vi "Disconnect SMU Resources from site - Site SMUs only.vi"(0 "TSM context":T1, 11 "error in":errorcluster) -> (4 "TSM context out":T1, 15 "error out":errorcluster)   [LabVIEW 2019]
doc: "This VI is used to disconnect SMU resources safely by preventing potetial OCP errors."
uses:
  <vilib>/NI_TestStand_SemiconductorModule/NI_TestStand_Semiconductor_Module.lvlibp/PinMap/General/SemiconductorModuleContext.ctl
  <instrlib>/niDCPower/nidcpower.llb/niDCPower Output Function.ctl
  <instrlib>/niDCPower/nidcpower.llb/niDCPower Sense.ctl
  <instrlib>/niDCPower/nidcpower.llb/niDCPower Source Mode.ctl
  TSM Context Data Access/Public/Properties/TestFlowID - Read.vi
  <vilib>/NI_TestStand_SemiconductorModule/NI_TestStand_Semiconductor_Module.lvlibp
  TSM Context Data Access/TSM Context Data Access.lvclass
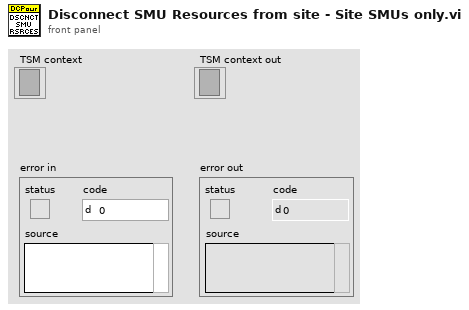
[diagram p1: front panel]
types:
  T1 = typedef "NI_TestStand_Semiconductor_Module.lvlibp/SemiconductorModuleContext.ctl" = refnum<k7>
  T2 = typedef "niDCPower Source Mode.ctl" = i32
  T3 = typedef "niDCPower Sense.ctl" = i32
  T4 = typedef "niDCPower Output Function.ctl" = i32
  T5 = typedef "TSM SSC DCPower.ctl" = cluster{"Pin Query Context":refnum<class "MultiplePinMultipleSessionQueryContext.lvclass">, "SSC":T6[], "Site Numbers":i32[], "Pins":T7[], "Pins Expanded":T9[]}
  T6 = typedef "SSC DCPower.ctl" = cluster{"Session":refnum<k15>, "Chan":string, "Channel List":string}
  T7 = typedef "TSM Pin Information.ctl" = cluster{"Pin":tag, "Type":T8, "Count":i32}
  T8 = typedef "TSM Pin Type Identifier.ctl" = enum8{"DUT Pin", "System Pin", "Pin Group", "Not Determined"}
  T9 = typedef "TSM Expanded Pin Information.ctl" = cluster{"Pin":tag, "Type":T8, "Index":i32}
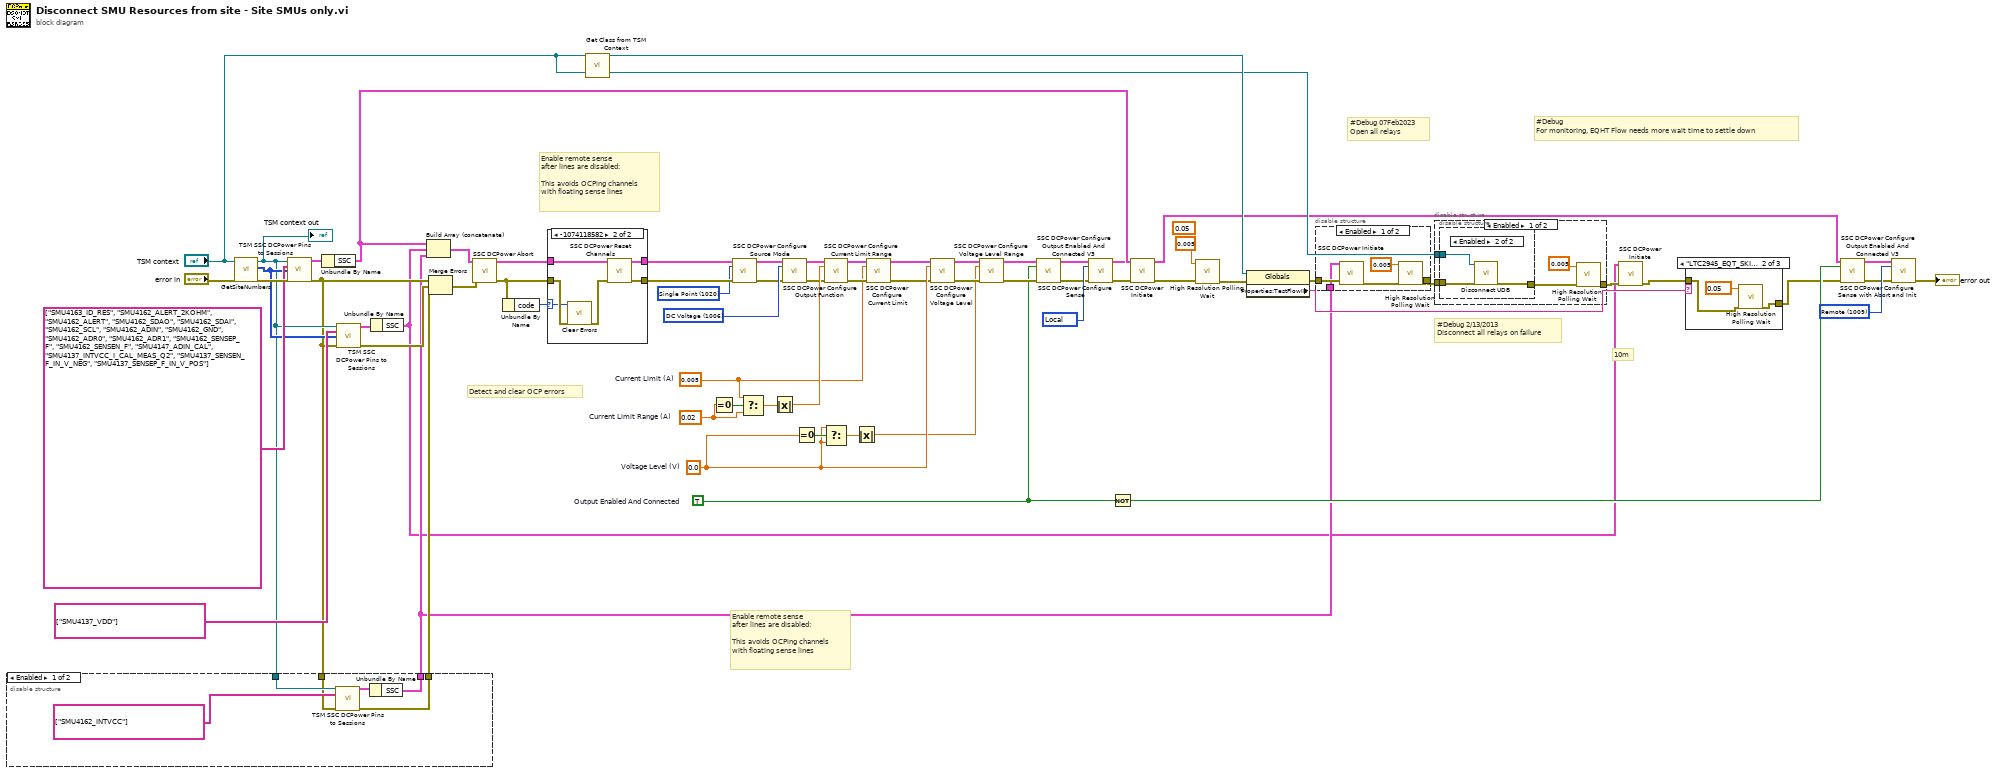
[diagram p0: block diagram]
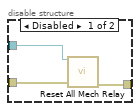
[diagram p2: hidden frame]
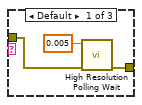
[diagram p6: hidden frame]
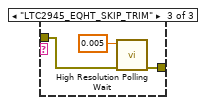
[diagram p7: hidden frame]
diagram:
  (unwired) 0.05 ("seconds to wait")
  w36 = T2 1020 items=["Single Point"=1020, "Sequence"=1021] ("Source Mode")
  w41 = T3 1009 items=["Local"=1008, "Remote"=1009] ("Sense")
  w43 = T3 1008 items=["Local"=1008, "Remote"=1009] ("Sense")
  w52 = T4 1006 items=["DC Voltage"=1006, "DC Current"=1007, "Pulse Voltage"=1049, "Pulse Current"=1050] ("Output Function")
  w51 = 0.005  # Current Limit (A)
  w49 = 0.0  # Voltage Level (V)
  w50 = 0.02  # Current Limit Range (A)
  w31 = TRUE  # Output Enabled And Connected
  # "10m"
  # "#Debug 2/13/2013\nDisconnect all relays on failure"
  # "#Debug 07Feb2023\nOpen all relays"
  # "#Debug\nFor monitoring, EQHT Flow needs more wait time to settle down"
  # "Enable remote sense\nafter lines are disabled:\n\nThis avoids OCPing channels\nwith floating sense lines"
  # "Enable remote sense\nafter lines are disabled:\n\nThis avoids OCPing channels\nwith floating sense lines"
  # "Detect and clear OCP errors"
  n1 = call <vilib>:"GetSiteNumbers.vi"("error in (no error)"="error in", "Semiconductor Module Context"="TSM context") -> ("error out"=w62:errorcluster, "Site Numbers"=w14:i32[], "Semiconductor Module Context Out"=w13:T1)  [unwired: 6 in, 1 out]
  "TSM context out" <- w13
  n2 = call "TSM SSC DCPower Pins to Sessions.vi"("TSM context"=w13, "Pins"=tag[] ["SMU4163_ID_RES", "SMU4162_ALERT_2KOHM", "SMU4162_ALERT", "SMU4162_SDAO", "SMU4162_SDAI", "SMU4162_SCL", "SMU4162_ADIN", "SMU4162_GND", "SMU4162_ADR0", "SMU4162_ADR1", "SMU4162_SENSEP_F", "SMU4162_SENSEN_F", "SMU4147_ADIN_CAL", "SMU4137_INTVCC_I_CAL_MEAS_Q2", "SMU4137_SENSEN_F_IN_V_NEG", "SMU4137_SENSEP_F_IN_V_POS"], "Site Numbers"=w14, "error in"=w62) -> ("DCPower TSM Out"=w64:T5, "error out"=w12:errorcluster)  [unwired: 10 in]
  n3 = disable-structure shown="Enabled" {
    disable-tunnel: w13 -> [w71 _]
    disable-tunnel: w12 -> [w69 _]
    disable-tunnel: [w68 _] -> w11
    disable-tunnel: [w67 _] -> w10
    frame Enabled {
      n4 = call "TSM SSC DCPower Pins to Sessions.vi"("TSM context"=w71, "Pins"=tag[] ["SMU4162_INTVCC"] ("Pin"), "error in"=w69) -> ("DCPower TSM Out"=w70:T5, "error out"=w68:errorcluster)  [unwired: 11 in]
      n5 = Unbundle By Name(w70) -> ("SSC"=w67:T6[])
    }
    frame Disabled {
    }
  }
  n6 = Unbundle By Name(w64) -> ("SSC"=w21:T6[])
  n7 = call "TSM SSC DCPower Pins to Sessions.vi"("TSM context"=w13, "Pins"=tag[] ["SMU4137_VDD"] ("Pin"), "Site Numbers"=w14, "error in"=w12) -> ("DCPower TSM Out"=w23:T5, "error out"=w25:errorcluster)  [unwired: 10 in]
  n8 = Unbundle By Name(w23) -> ("SSC"=w2:T6[])
  n9 = Build Array (concatenate)(w21, w2, w10) -> (w22:T6[])
  n10 = Merge Errors(w12, w25, w11) -> (w24:errorcluster)
  n11 = call "SSC DCPower Abort.vi"("DCPower SSC in"=w22, "error in"=w24) -> ("DCPower SSC out"=w63:T6[], "error out"=w65:errorcluster)  [unwired: 12 in]
  n12 = Unbundle By Name(w65) -> ("code"=w66:i32)
  n13 = case shown="-1074118582" w66 {
    selector: w66 -> [_ w77]
    tunnel: [w74 w79] -> w40
    tunnel: w65 -> [w74 w80]
    tunnel: w63 -> [w73 w76]
    tunnel: [w73 w75] -> w39
    frame Default {
    }
    frame -1074118582 {
      n14 = call <vilib>:"Clear Errors.vi"("error in (no error)"=w80, "specific error code to clear (0: all)"=w77) -> ("error out"=w78:errorcluster)  [unwired: 4 in, 1 out]
      n15 = call "SSC DCPower Reset Channels.vi"("DCPower SSC in"=w76, "error in"=w78) -> ("DCPower SSC out"=w75:T6[], "error out"=w79:errorcluster)  [unwired: 12 in]
    }
  }
  n16 = call "Get Class from TSM Context.vi"("TSM Context"="TSM context") -> ("Global Memory Class"=w18:refnum<class "TSM Context Data Access.lvclass">)  [unwired: 14 in]
  n17 = Equal To 0?(x=w50) -> (x = 0?=w60:bool)
  n18 = call "SSC DCPower Configure Source Mode.vi"("DCPower SSC in"=w39, "Source Mode"=w36, "error in"=w40) -> ("DCPower SSC out"=w37:T6[], "error out"=w38:errorcluster)  [unwired: 11 in]
  n19 = Select(t=w51, s=w60, f=w50) -> (s? t:f=w59:dbl)
  n20 = Absolute Value(x=w59) -> (abs(x)=w61:dbl)
  n21 = call "SSC DCPower Configure Output Function.vi"("DCPower SSC in"=w37, "Output Function"=w52, "error in"=w38) -> ("DCPower SSC out"=w53:T6[], "error out"=w54:errorcluster)  [unwired: 11 in]
  n22 = Equal To 0?(x=w49) -> (x = 0?=w57:bool)
  n23 = call "SSC DCPower Configure Current Limit Range.vi"("DCPower SSC in"=w53, "Current Limit Range (A)"=w61, "error in"=w54) -> ("DCPower SSC out"=w55:T6[], "error out"=w56:errorcluster)  [unwired: 11 in]
  n24 = Select(t=w49, s=w57, f=w49) -> (s? t:f=w58:dbl)
  n25 = Absolute Value(x=w58) -> (abs(x)=w44:dbl)
  n26 = call "SSC DCPower Configure Current Limit.vi"("DCPower SSC in"=w55, "Current Limit (A)"=w51, "error in"=w56) -> ("DCPower SSC out"=w47:T6[], "error out"=w48:errorcluster)  [unwired: 11 in]
  n27 = call "SSC DCPower Configure Voltage Level.vi"("DCPower SSC in"=w47, "Voltage Level (V)"=w49, "error in"=w48) -> ("DCPower SSC out"=w45:T6[], "error out"=w46:errorcluster)  [unwired: 11 in]
  n28 = call "SSC DCPower Configure Voltage Level Range.vi"("DCPower SSC in"=w45, "Voltage Level Range (V)"=w44, "error in"=w46) -> ("DCPower SSC out"=w32:T6[], "error out"=w33:errorcluster)  [unwired: 11 in]
  n29 = call "SSC DCPower Configure Output Enabled And Connected V3.vi"("DCPower SSC in"=w32, "Output Enabled And Connected"=w31, "error in"=w33) -> ("DCPower SSC out"=w29:T6[], "error out"=w30:errorcluster)  [unwired: 11 in]
  n30 = call "SSC DCPower Configure Sense.vi"("DCPower SSC in"=w29, "Sense"=w43, "error in"=w30) -> ("DCPower SSC out"=w8:T6[], "error out"=w42:errorcluster)  [unwired: 11 in]
  n31 = Not(x=w31) -> (.not. x?=w16:bool)
  n32 = call "SSC DCPower Initiate.vi"("DCPower SSC in"=w21, "error in"=w42) -> ("error out"=w7:errorcluster)  [unwired: 12 in, 1 out]
  n33 = call <vilib>:"High Resolution Polling Wait.vi"("error in (no error)"=w7, "seconds to wait"=0.005) -> ("error out"=w6:errorcluster)  [unwired: 9 in]
  n34 = property class="Globals"(reference=w18, error in=w6) -> (error out=w19:errorcluster, "Properties:TestFlowID"=w20:string)  [unwired: 1 out]
  n35 = disable-structure shown="Enabled" {
    disable-tunnel: w19 -> [w85 w86]
    disable-tunnel: w10 -> [w84 _]
    disable-tunnel: [w82 w86] -> w9
    frame Enabled {
      n36 = call "SSC DCPower Initiate.vi"("DCPower SSC in"=w84, "error in"=w85) -> ("error out"=w83:errorcluster)  [unwired: 12 in, 1 out]
      n37 = call <vilib>:"High Resolution Polling Wait.vi"("error in (no error)"=w83, "seconds to wait"=0.005) -> ("error out"=w82:errorcluster)  [unwired: 9 in]
    }
    frame Disabled {
    }
  }
  n38 = disable-structure shown="Enabled" {
    disable-tunnel: "TSM context" -> [w91 _]
    disable-tunnel: w9 -> [w90 w98]
    disable-tunnel: [w88 w98] -> w3
    frame Enabled {
      n39 = disable-structure shown="Enabled" {
        disable-tunnel: w90 -> [w94 w97]
        disable-tunnel: [w93 w96] -> w89
        disable-tunnel: w91 -> [w92 w95]
        frame Disabled {
          n40 = call "Reset All Mech Relay.vi"("TSM Context"=w92, "error in (no error)"=w94) -> ("error out"=w93:errorcluster)  [unwired: 13 in]
        }
        frame Enabled {
          n41 = call "Disconnect UDB.vi"("error in (no error)"=w97, "Semiconductor Module Context"=w95) -> ("error out"=w96:errorcluster)  [unwired: 9 in]
        }
      }
      n42 = call <vilib>:"High Resolution Polling Wait.vi"("error in (no error)"=w89, "seconds to wait"=0.005) -> ("error out"=w88:errorcluster)  [unwired: 9 in]
    }
    frame Disabled {
    }
  }
  n43 = call "SSC DCPower Initiate.vi"("DCPower SSC in"=w2, "error in"=w3) -> ("error out"=w1:errorcluster)  [unwired: 12 in, 1 out]
  n44 = case shown="\"LTC2945_EQT_SKIP_TRIM\"" w20 {
    tunnel: [w100 w102 w106] -> w4
    tunnel: w1 -> [w99 w103 w105]
    frame Default {
      n45 = call <vilib>:"High Resolution Polling Wait.vi"("error in (no error)"=w99, "seconds to wait"=0.005) -> ("error out"=w100:errorcluster)  [unwired: 9 in]
    }
    frame "LTC2945_EQT_SKIP_TRIM" {
      n46 = call <vilib>:"High Resolution Polling Wait.vi"("error in (no error)"=w103, "seconds to wait"=0.05) -> ("error out"=w102:errorcluster)  [unwired: 9 in]
    }
    frame "LTC2945_EQHT_SKIP_TRIM" {
      n47 = call <vilib>:"High Resolution Polling Wait.vi"("error in (no error)"=w105, "seconds to wait"=0.005) -> ("error out"=w106:errorcluster)  [unwired: 9 in]
    }
  }
  n48 = call "SSC DCPower Configure Output Enabled And Connected V3.vi"("DCPower SSC in"=w8, "Output Enabled And Connected"=w16, "error in"=w4) -> ("DCPower SSC out"=w27:T6[], "error out"=w28:errorcluster)  [unwired: 11 in]
  n49 = call "SSC DCPower Configure Sense with Abort and Init.vi"("DCPower SSC in"=w27, "Sense"=w41, "error in"=w28) -> ("error out"=→"error out":errorcluster)  [unwired: 11 in, 1 out]
